vi "FGV-GlobalEventRef.vi"(6 "Create(F)":bool, 8 "error in (no error)":errorcluster) -> (0 "error out":errorcluster, 3 "CSM Global Log Event":refnum<user-event>)   [LabVIEW 2020, in "Communicable State Machine.lvlib"]
uses:
  Communicable State Machine.lvlib
  _CSM_GlobalLog_MSG.ctl
  _CSM_Response Source Message.ctl
  _CSM_GlobalLog_MSG_TYPE.ctl
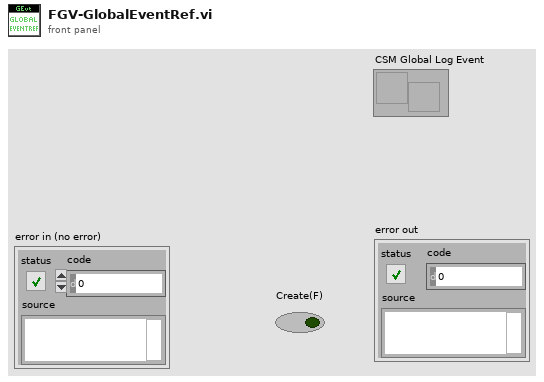
[diagram p1: front panel]
types:
  T1 = typedef "Communicable State Machine.lvlib/_CSM_GlobalLog_MSG.ctl" = cluster{"Name(\"\" to use uuid)":string, "Current State":string, "Arguments":string, "Source Message":T2, "Source Module":string, "Complete(T)/Start(F)":bool, "LogType":T3}
  T2 = typedef "Communicable State Machine.lvlib/_CSM_Response Source Message.ctl" = cluster{"‘State":string, "’Arguments":string, "’Error":errorcluster}
  T3 = typedef "Communicable State Machine.lvlib/_CSM_GlobalLog_MSG_TYPE.ctl" = enum16{"User Log", "State Change", "Status", "Interrupt", "Register", "Unregister", "Error Log", "Module Created", "Module Destroyed"}
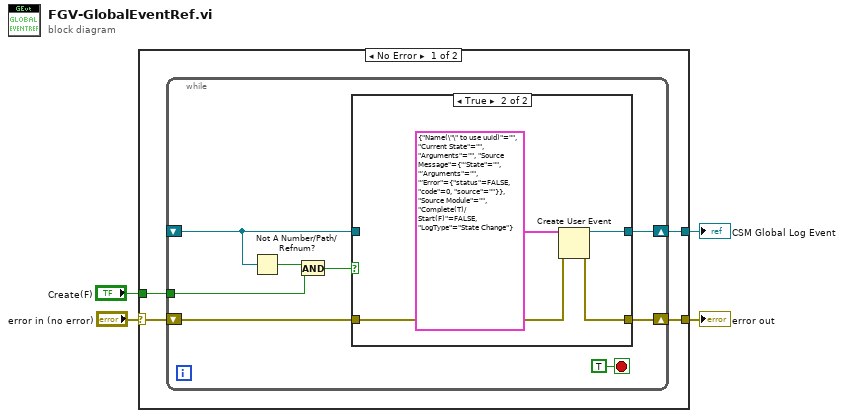
[diagram p0: block diagram]
diagram:
  n1 = case shown="No Error" "error in (no error)" {
    selector: "error in (no error)" -> [w7 w23]
    tunnel: [w8 _] -> w4
    tunnel: [w6 w23] -> w2
    tunnel: "Create(F)" -> [w5 _]
    frame No Error {
      n2 = while {
        shift-right: [w14] -> w6
        shift-left: w7 -> [w15]
        shift-right: [w16] -> w8
        shift-left: _ -> [w12]
        tunnel: w5 -> [w9]
        stop <- TRUE stop-if-true
        n3 = Not A Number/Path/Refnum?(number/path/refnum=w12) -> (NaN/Path/Refnum?=w10:bool)
        n4 = And(x=w10, y=w9) -> (x .and. y?=w11:bool)
        n5 = case shown="True" w11 {
          tunnel: [w18 w21] -> w16
          tunnel: w15 -> [w17 w19]
          tunnel: [w17 w20] -> w14
          tunnel: w12 -> [w18 _]
          frame False {
          }
          frame True {
            n6 = Create User Event(user event datatype=T1 {"Name(\"\" to use uuid)"="", "Current State"="", "Arguments"="", "Source Message"={"‘State"="", "’Arguments"="", "’Error"={"status"=FALSE, "code"=0, "source"=""}}, "Source Module"="", "Complete(T)/Start(F)"=FALSE, "LogType"=enum."State Change"} ("Cross JKI State Machine Data"), error in=w19) -> (user event=w21:refnum<user-event>, error out=w20:errorcluster)
          }
        }
      }
    }
    frame Error {
    }
  }
  "CSM Global Log Event" <- w4
  "error out" <- w2
